vi "(SubVI)System Command_Trig GPIO Control.vi"(8 "error in (no error)":errorcluster caption="에러 입력(에러 없음)", 11 "Trig_Ctrl":T1={"1st Trig"={"Trigger"=FALSE, "Low"=1, "High"=1}, "2nd Trig"={"Trigger"=FALSE, "Low"=1, "High"=1}, "3rd Trig"={"Trigger"=FALSE, "Low"=1, "High"=1}, "4th Trig"={"Trigger"=FALSE, "Low"=1, "High"=1}} {"4th Trig"."High" min=1; "4th Trig"."Low" min=1; "3rd Trig"."High" min=1; "3rd Trig"."Low" min=1; "2nd Trig"."High" min=1; "2nd Trig"."Low" min=1; "1st Trig"."High" min=1; "1st Trig"."Low" min=1}) -> (0 "error out":errorcluster caption="에러 출력")   [LabVIEW 2020]
uses:
  Controls/(Ctrl)System Command_Trig GPIO Control.ctl
  Serial/Instance VIs/(SubVI)Serial_Write.vi
panel:
  # "Trigger"
  # "L (us)"
  # "H (us)"
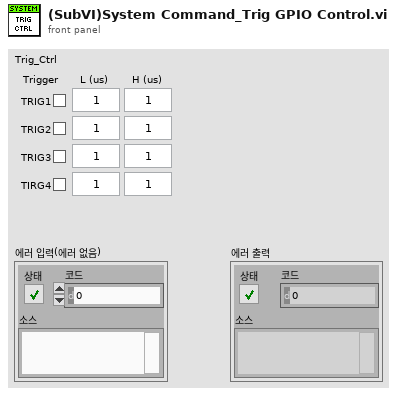
[diagram p1: front panel]
types:
  T1 = typedef "(Ctrl)System Command_Trig GPIO Control.ctl" = cluster{"1st Trig":cluster{"Trigger":bool, "Low":u16, "High":u16}, "2nd Trig":cluster{"Trigger":bool, "Low":u16, "High":u16}, "3rd Trig":cluster{"Trigger":bool, "Low":u16, "High":u16}, "4th Trig":cluster{"Trigger":bool, "Low":u16, "High":u16}}
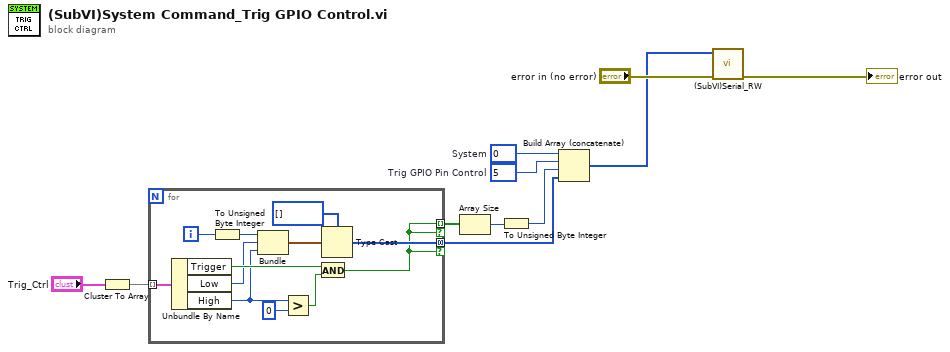
[diagram p0: block diagram]
diagram:
  w10 = u8 5  # Trig GPIO Pin Control
  w11 = u8 0  # System
  n1 = Cluster To Array(cluster="Trig_Ctrl") -> (array=w5:cluster{"Trigger":bool, "Low":u16, "High":u16}[])
  n2 = for {
    tunnel: w5 -> [w22] mode=indexing
    tunnel: [w21] -> w4 mode=concatenating if=w12
    tunnel: [w12] -> w3 mode=indexing if=w12
    i -> [w17]
    n3 = Unbundle By Name(w22) -> ("Trigger"=w18:bool, "Low"=w15:u16, "High"=w14:u16)
    n4 = To Unsigned Byte Integer(number=w17) -> (unsigned 8bit integer=w16:u8)
    n5 = Bundle(w16, "Low"=w15, "High"=w14) -> (w13:cluster{u8, "Low":u16, "High":u16})  [unwired: 1 in]
    n6 = Greater?(x=w14, y=u16 0) -> (0:w19:bool)
    n7 = And(x=w18, y=w19) -> (x .and. y?=w12:bool)
    n8 = Type Cast(type=u8[] [], x=w13) -> (*(type *) &x=w21:u8[])
  }
  n9 = Array Size(array=w3) -> (size(s)=w1:i32)
  n10 = To Unsigned Byte Integer(number=w1) -> (unsigned 8bit integer=w2:u8)
  n11 = Build Array (concatenate)(w11, w10, w2, w4) -> (w7:u8[])
  n12 = call-poly "(SubVI)Serial_RW.vi"("error in (no error)"="error in (no error)", "Data to Write"=w7) -> ("error out"=→"error out":errorcluster)  [unwired: 9 in]
